vi "DialogGetNameAndClass.vi"(8 "error in (no error)":errorcluster) -> (0 "error out":errorcluster, 1 "Cancelled":bool, 2 "Class":string, 3 "Name":string)   [LabVIEW 2022 SP3, in "Object_Editor.lvlib" / "Object_Editor.lvclass"]
uses:
  Object_Editor.lvclass
  <userlib>/_OpenG.lib/string/string.llb/Trim Whitespace (String)__ogtk.vi
  <vilib>/regexp/Match Regular Expression.xnode
panel:
  in  "Cancel":bool
  in  "OK":bool
  in  "Class":i32(listbox)
  in  "Name":string
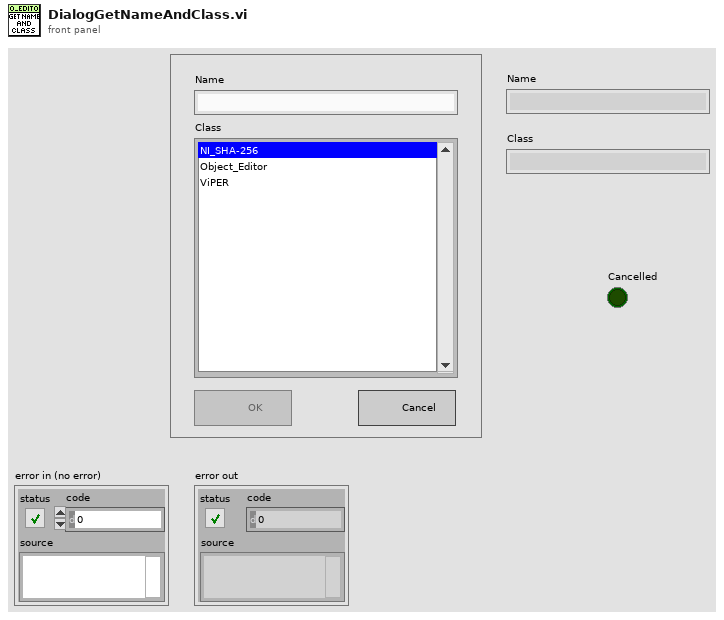
[diagram p1: front panel]
types:
  T1 = enum8{"Enabled", "Disabled", "Disabled and Grayed Out"}
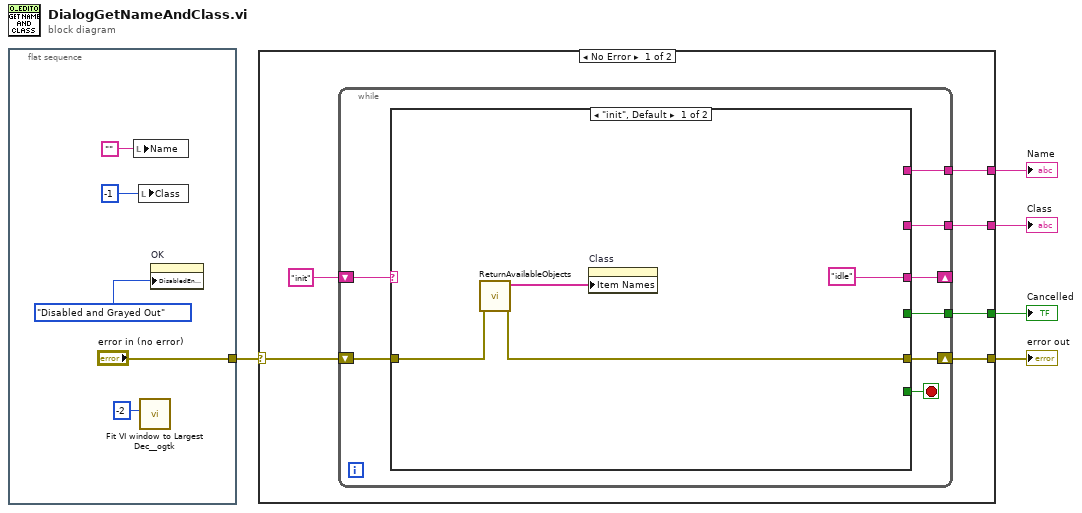
[diagram p0: block diagram]
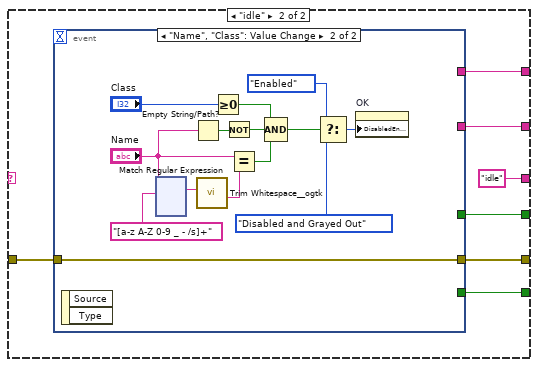
[diagram p2: hidden frame]
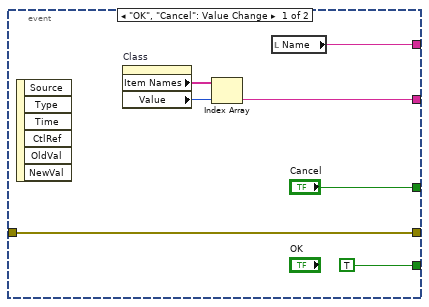
[diagram p3: hidden frame]
diagram:
  n1 = flat-sequence {
    tunnel: ["error in (no error)"] -> w5
    frame #0 {
      n2 = local write "Name"("") -> ()
      n3 = local write "Class"(-1 ("Class")) -> ()
      n4 = call <userlib>:"Fit VI window to Largest Dec__ogtk.vi"("border spacing (2 px)"=-2) -> ()  [unwired: 5 in, 2 out]
      n5 = property on="OK" class="Bool"("DisabledEnum"=T1."Disabled and Grayed Out" ("Disabled")) -> ()  [unwired: 2 in, 2 out]
    }
  }
  n6 = case shown="No Error" w5 {
    selector: w5 -> [w16 w174]
    tunnel: [w15 w174] -> w4
    tunnel: [w14 _] -> w3
    tunnel: [w12 _] -> w2
    tunnel: [w11 _] -> w1
    frame No Error {
      n7 = while {
        shift-right: [w23] -> w15
        shift-left: w16 -> [w24]
        tunnel: [w21] -> w14
        shift-right: [w19] -> _
        shift-left: "init" -> [w20]
        tunnel: [w18] -> w12
        tunnel: [w17] -> w11
        stop <- w22 stop-if-true
        n8 = case shown="\"init\", Default" w20 {
          tunnel: w24 -> [w27 w35]
          tunnel: [w26 w34] -> w23
          tunnel: [_ w33] -> w22
          tunnel: [_ w32] -> w21
          tunnel: ["idle" "idle"] -> w19
          tunnel: [_ w30] -> w18
          tunnel: [_ w29] -> w17
          frame "init", Default {
            n9 = call "ReturnAvailableObjects.vi"("error in (no error)"=w27) -> ("error out"=w26:errorcluster, "Output Array"=w25:string[])  [unwired: 9 in]
            n10 = property on="Class" class="LstBox (strict)"("Item Names"=w25) -> ()  [unwired: 2 in, 2 out]
          }
          frame "idle" {
            n11 = event shown="[1] \"Name\", \"Class\": Value Change" {
              selector: _ -> [_ _]
              dyn-events: _ -> [_ _]
              timeout: _ -> [_ _]
              tunnel: w35 -> [w42 w50]
              tunnel: [w42 w50] -> w34
              tunnel: [TRUE ("OK") _] -> w33
              tunnel: ["Cancel" _] -> w32
              tunnel: [w39 _] -> w30
              tunnel: [w36 _] -> w29
              event "OK", "Cancel": Value Change {
                n12 = event-data() -> ()  [unwired: 1 in, 6 out]
                n13 = property on="Class" class="LstBox (strict)"() -> ("Item Names"=w38:string[], "Value"=w37:i32)  [unwired: 2 in, 2 out]
                n14 = Index Array(array=w38, index=w37) -> (element=w36:string)
                n15 = local read "Name"() -> (w39:string)
              }
              event "Name", "Class": Value Change {
                n16 = event-data() -> ()  [unwired: 1 in, 2 out]
                n17 = xnode "Match Regular Expression"("input string"="Name", "regular expression"="[a-z A-Z 0-9 _ - /s]+") -> ("whole match"=w55:string)  [unwired: 4 in, 4 out]
                n18 = Empty String/Path?(string/path="Name") -> (empty?=w47:bool)
                n19 = call-poly <userlib>:"Trim Whitespace__ogtk.vi"("String in"=w55) -> ("String out"=w54:string)  [unwired: 6 in]
                n20 = Greater Or Equal To 0?(x="Class") -> (x >= 0?=w46:bool)
                n21 = Not(x=w47) -> (.not. x?=w45:bool)
                n22 = Equal?(x="Name", y=w54) -> (x = y?=w44:bool)
                n23 = Compound Arithmetic op=AND(w46, w45, w44) -> (w43:bool)
                n24 = Select(t=T1."Enabled" ("Disabled"), s=w43, f=T1."Disabled and Grayed Out" ("Disabled")) -> (s? t:f=w51:T1)
                n25 = property on="OK" class="Bool"("DisabledEnum"=w51) -> ()  [unwired: 2 in, 2 out]
              }
            }
          }
        }
      }
    }
    frame Error {
    }
  }
  "error out" <- w4
  "Name" <- w2
  "Class" <- w1
  "Cancelled" <- w3
